vi "globlas.vi"() -> ()   [LabVIEW 2019]
panel:
  out "BAT 2 V":dbl
  out "BAT 1 V":dbl
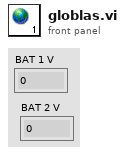
[diagram p1: front panel]
diagram:
